vi "Initialization VI.vi"(8 "error in (no error)":errorcluster, 10 "Custom XML":string, 11 "Device Item Ref in":T1 format="%.0x") -> (0 "error out":errorcluster, 3 "Device Item Ref out":T1 format="%.0x")   [LabVIEW 2019, in "UDP-Custom-Device System Explorer.lvlib"]
uses:
  UDP-Custom-Device System Explorer.lvlib
  <vilib>/NI VeriStand/Custom Device API/Custom Device Item Ref.ctl
  <vilib>/NI VeriStand/Custom Device API/Custom Device API.lvlib
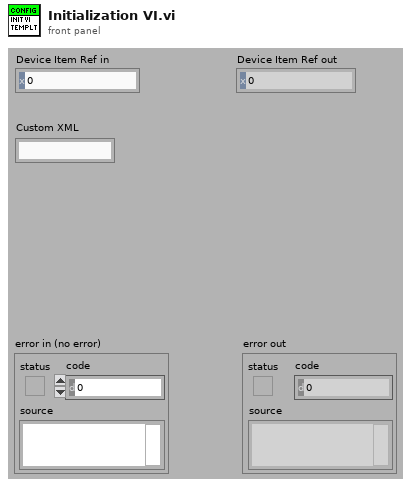
[diagram p1: front panel]
types:
  T1 = typedef "Custom Device API.lvlib/Custom Device Item Ref.ctl" = u64
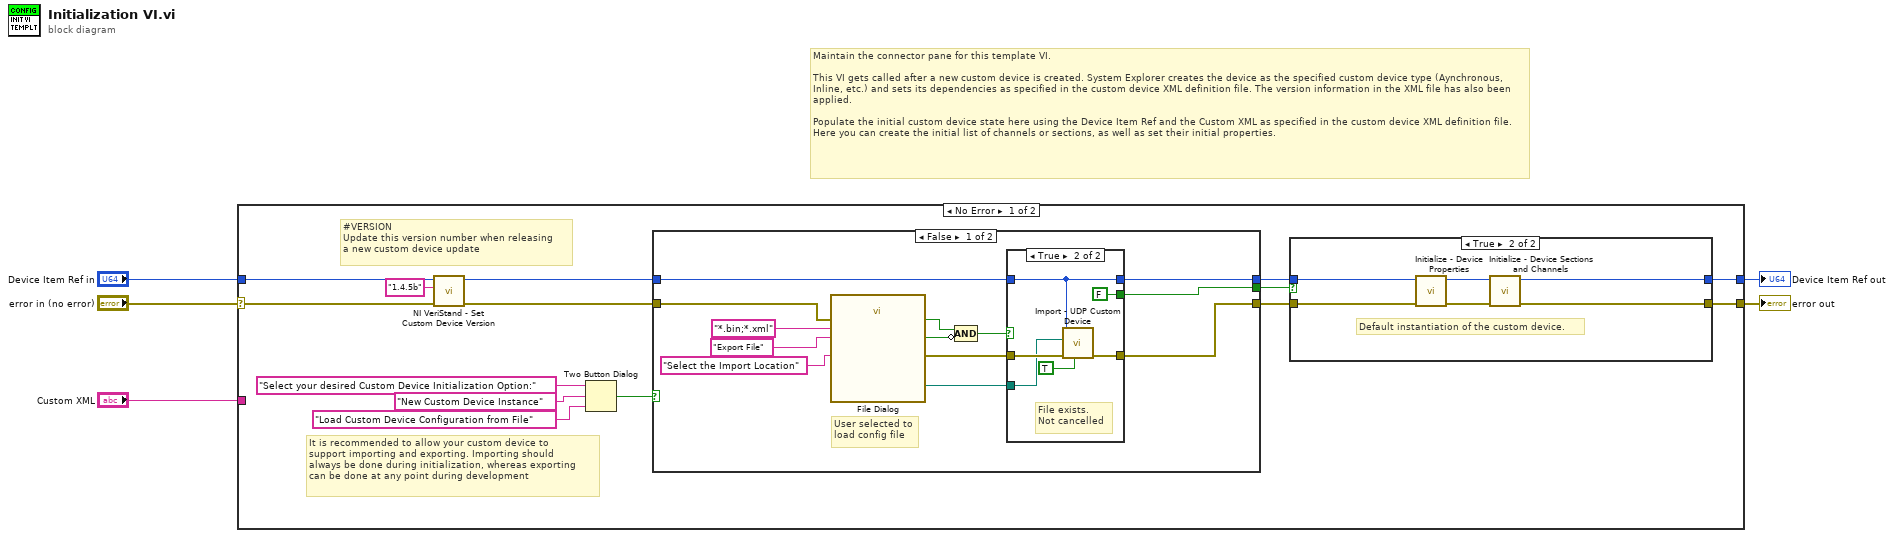
[diagram p0: block diagram]
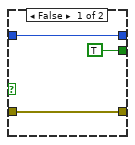
[diagram p3: hidden frame]
diagram:
  # "Maintain the connector pane for this template VI.\n\nThis VI gets called after a new custom device is created. System Explorer creates the device as the specified custom device type (Aynchronous, Inline, etc.) and sets its dependencies as specified in the custom device XML definition file. The version information in the XML file has also been applied.\n\nPopulate the initial custom device state here using the Device Item Ref and the Custom XML as specified in the custom device XML definition file. Here you can create the initial list of channels or sections, as well as set their initial properties."
  n1 = case shown="No Error" "error in (no error)" {
    selector: "error in (no error)" -> [w8 w54]
    tunnel: [w12 w54] -> w5
    tunnel: [w11 w53] -> w3
    tunnel: "Device Item Ref in" -> [w10 w53]
    tunnel: "Custom XML" -> [_ _]
    frame No Error {
      # "#VERSION\nUpdate this version number when releasing\na new custom device update"
      # "It is recommended to allow your custom device to\nsupport importing and exporting. Importing should\nalways be done during initialization, whereas exporting\ncan be done at any point during development"
      n2 = call <vilib>:"NI VeriStand - Set Custom Device Version.vi"("error in (no error)"=w8, "Value"="1.4.5b", "Device Ref in"=w10) -> ("error out"=w7:errorcluster, "Device Ref out"=w9:T1)  [unwired: 7 in]
      n3 = Two Button Dialog(message="Select your desired Custom Device Initialization Option:", 1:"Load Custom Device Configuration from File" ("F button name (\"Cancel\")"), 2:"New Custom Device Instance" ("T button name (\"OK\")")) -> (T button?=w16:bool)
      n4 = case shown="False" w16 {
        selector: w16 -> [_ w50]
        tunnel: w9 -> [w34 w52]
        tunnel: [w33 w52] -> w15
        tunnel: w7 -> [w28 w51]
        tunnel: [w35 w51] -> w13
        tunnel: [w31 w50] -> w14
        frame False {
          # "User selected to\nload config file"
          n5 = call "File Dialog"("prompt"="Select the Import Location", "error in"=w28, "pattern (all files)"="*.bin;*.xml", "pattern label"="Export File") -> ("selected path"=w32:path, "exists"=w39:bool, "cancelled"=w38:bool, "error out"=w36:errorcluster)  [unwired: 8 in]
          n6 = Compound Arithmetic op=AND(w39, invert w38) -> (w37:bool)
          n7 = case shown="True" w37 {
            tunnel: w36 -> [w42 w48]
            tunnel: [w42 w47] -> w35
            tunnel: [w43 w49] -> w33
            tunnel: w34 -> [w43 w49]
            tunnel: w32 -> [_ w46]
            tunnel: [TRUE FALSE] -> w31
            frame False {
            }
            frame True {
              # "File exists.\nNot cancelled"
              n8 = call "Import - UDP Custom Device.vi"("New CD?"=TRUE, "error in (no error)"=w48, "Target File"=w46, "Device Item Ref in"=w49) -> ("error out"=w47:errorcluster)  [unwired: 7 in]
            }
          }
        }
        frame True {
          # "User selected new\ncustom device. Do\nnothing in this case\nand handle new\ngeneration in the\nnext case structure"
        }
      }
      n9 = case shown="True" w14 {
        tunnel: w15 -> [w21 w27]
        tunnel: w13 -> [w20 w26]
        tunnel: [w20 w24] -> w12
        tunnel: [w21 w23] -> w11
        frame False {
          # "User selected to import from configuration"
        }
        frame True {
          # "Default instantiation of the custom device."
          n10 = call "Initialize - Device Properties.vi"("error in (no error)"=w26, "Device Item Ref in"=w27) -> ("error out"=w25:errorcluster, "Item Ref out"=w22:T1)  [unwired: 8 in]
          n11 = call "Initialize - Device Sections and Channels.vi"("error in (no error)"=w25, "Item Ref out"=w22) -> ("error out"=w24:errorcluster, "Parent Ref out"=w23:T1)  [unwired: 8 in]
        }
      }
    }
    frame Error {
    }
  }
  "error out" <- w5
  "Device Item Ref out" <- w3
